vi "Lockin_on_waveform.vi"(9 "Frequency":dbl, 10 "waveform in":waveform(dbl), 11 "Number of Sines":dbl) -> (2 "Phase":waveform(dbl), 3 "Magnitude":waveform(dbl))   [LabVIEW 2015]
uses:
  <vilib>/Waveform/WDTOps.llb/WDT Get Waveform Time Array DBL.vi
  <vilib>/Analysis/NI_AALPro.lvlib
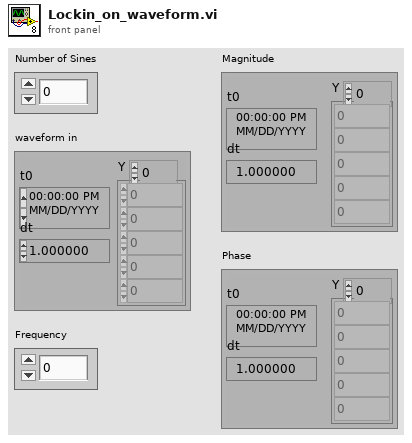
[diagram p1: front panel]
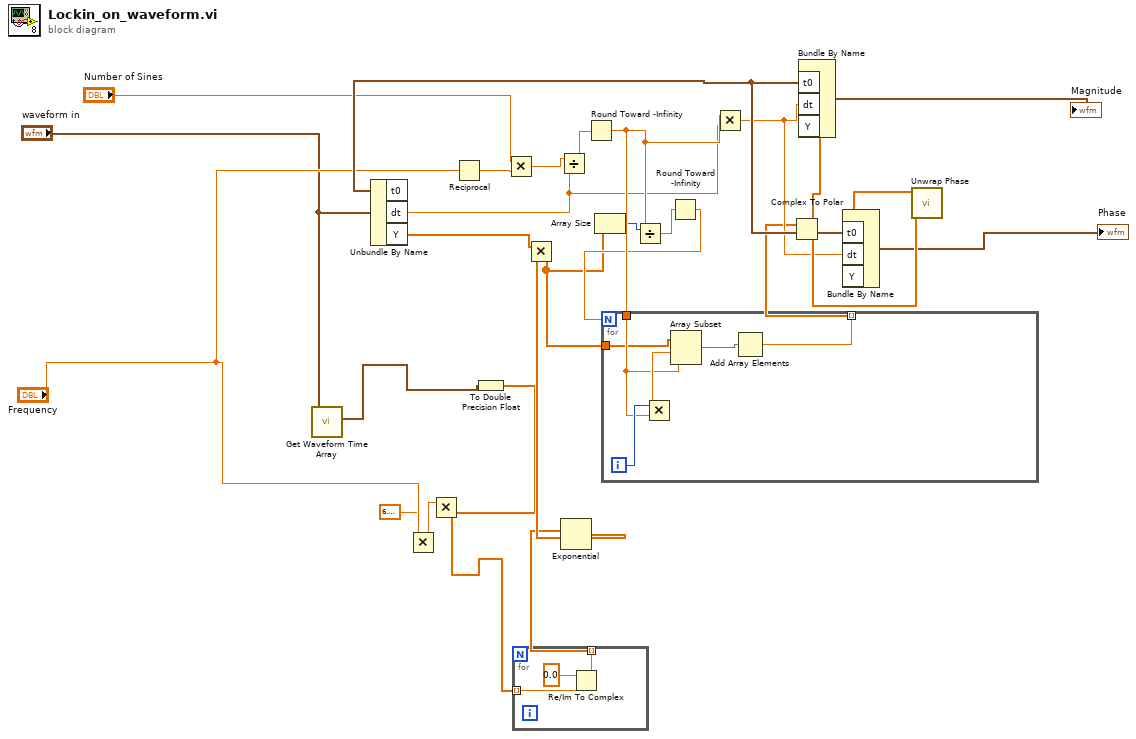
[diagram p0: block diagram]
diagram:
  n1 = call-poly <vilib>:"Get Waveform Time Array.vi"("waveform in"="waveform in") -> ("X array"=w1:timestamp[])  [unwired: 9 in, 1 out]
  n2 = Unbundle By Name("waveform in") -> ("t0"=w26:timestamp, "dt"=w20:dbl, "Y"=w9:dbl[])
  n3 = Multiply(x=6.283185307179586, y="Frequency") -> (x*y=w3:dbl)
  n4 = Reciprocal(x="Frequency") -> (1/x=w16:dbl)
  n5 = To Double Precision Float(number=w1) -> (double precision float=w4:dbl[])
  n6 = Multiply(x=w3, y=w4) -> (x*y=w5:dbl[])
  n7 = Multiply(x="Number of Sines", y=w16) -> (x*y=w18:dbl)
  n8 = for {
    tunnel: w5 -> [w31] mode=indexing
    tunnel: [w29] -> w6 mode=indexing
    n9 = Re/Im To Complex(1:w31, 2:0.0 ("x")) -> (0:w29:cdb)
  }
  n10 = Divide(x=w18, y=w20) -> (x/y=w19:dbl)
  n11 = Exponential(1:w6) -> (0:w8:cdb[])
  n12 = Multiply(x=w9, y=w8) -> (x*y=w10:cdb[])
  n13 = Round Toward -Infinity(1:w19) -> (0:w21:dbl)
  n14 = Array Size(array=w10) -> (size(s)=w11:i32)
  n15 = Divide(x=w11, y=w21) -> (x/y=w12:dbl)
  n16 = Round Toward -Infinity(1:w12) -> (0:w13:dbl)
  n17 = for {
    N: w13 -> [_]
    tunnel: w10 -> [w34]
    tunnel: w21 -> [w35]
    tunnel: [w32] -> w14 mode=indexing
    i -> [w37]
    n18 = Multiply(x=w37, y=w35) -> (x*y=w36:dbl)
    n19 = Array Subset(array=w34, index=w36, length=w35) -> (w33:cdb[])
    n20 = Add Array Elements(numeric array=w33) -> (sum=w32:cdb)
  }
  n21 = Multiply(x=w21, y=w20) -> (x*y=w25:dbl)
  n22 = Complex To Polar(r * e^(i*theta)=w14) -> (r=w22:dbl[], theta=w27:dbl[])
  n23 = Bundle By Name("t0"=w26, "dt"=w25, "Y"=w22) -> (→"Magnitude":waveform(dbl))  [unwired: 1 in]
  n24 = call <vilib>:"Unwrap Phase.vi"("Phase"=w27) -> ("Unwrapped Phase"=w28:dbl[])  [unwired: 9 in, 1 out]
  n25 = Bundle By Name("t0"=w26, "dt"=w25, "Y"=w28) -> (→"Phase":waveform(dbl))  [unwired: 1 in]
